vi "RB2 base station main 3.vi"() -> ()   [LabVIEW 2012]
uses:
  <vilib>/userdefined/High Color/IMAQdx.ctl
  <vilib>/vision/driver/NI_Vision_Acquisition_Software.lvlib
panel:
  out "Running?":bool
  out "All found?":bool
  in  "Data sent":string
  out "error out":errorcluster
  out "Image":T1(plugin-control)
  in  "stop":bool
  in  "Session In":T2="cam0"
  # "The Point Grey camera settings should be:\nAuto Exposure      Auto\nBrightness             Auto\nGain                       Auto\nFrame Rate           Auto\nShutter                  Auto\n\nThese values are programmed into this VI"
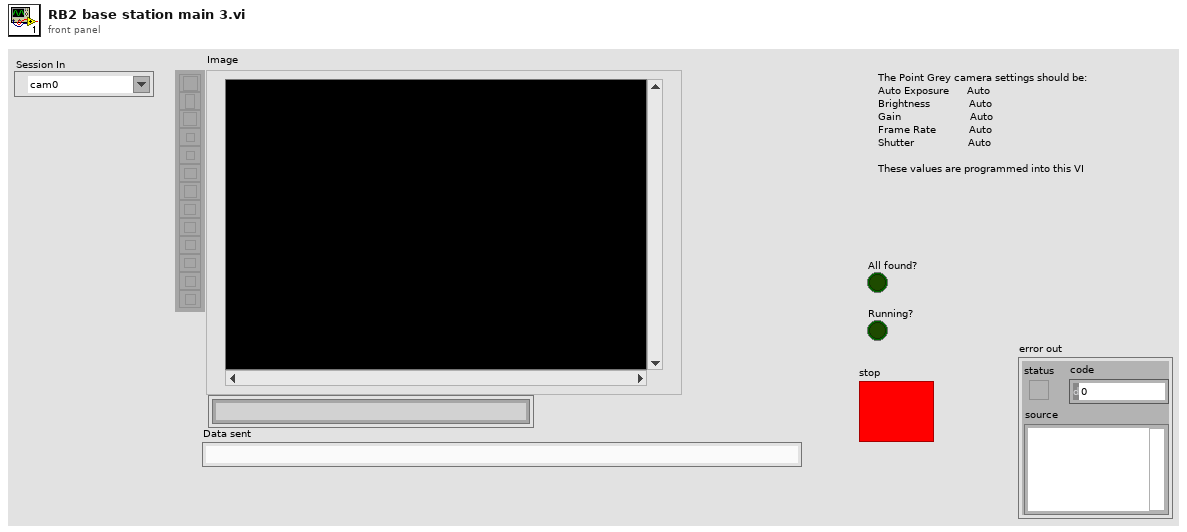
[diagram p1: front panel]
types:
  T1 = typedef "IMAQ Image.ctl" = refnum<image>
  T2 = typedef "IMAQdx.ctl" = refnum<k21>
  T3 = typedef "Image Type" = u32
  T4 = cluster{"String":string, "Pos. X":i32, "Pos. Y":i32, bool}[]
  T5 = cluster{"Pos. X":i32, "Pos. Y":i32, "Radius":i32, "Core Area":i32}[]
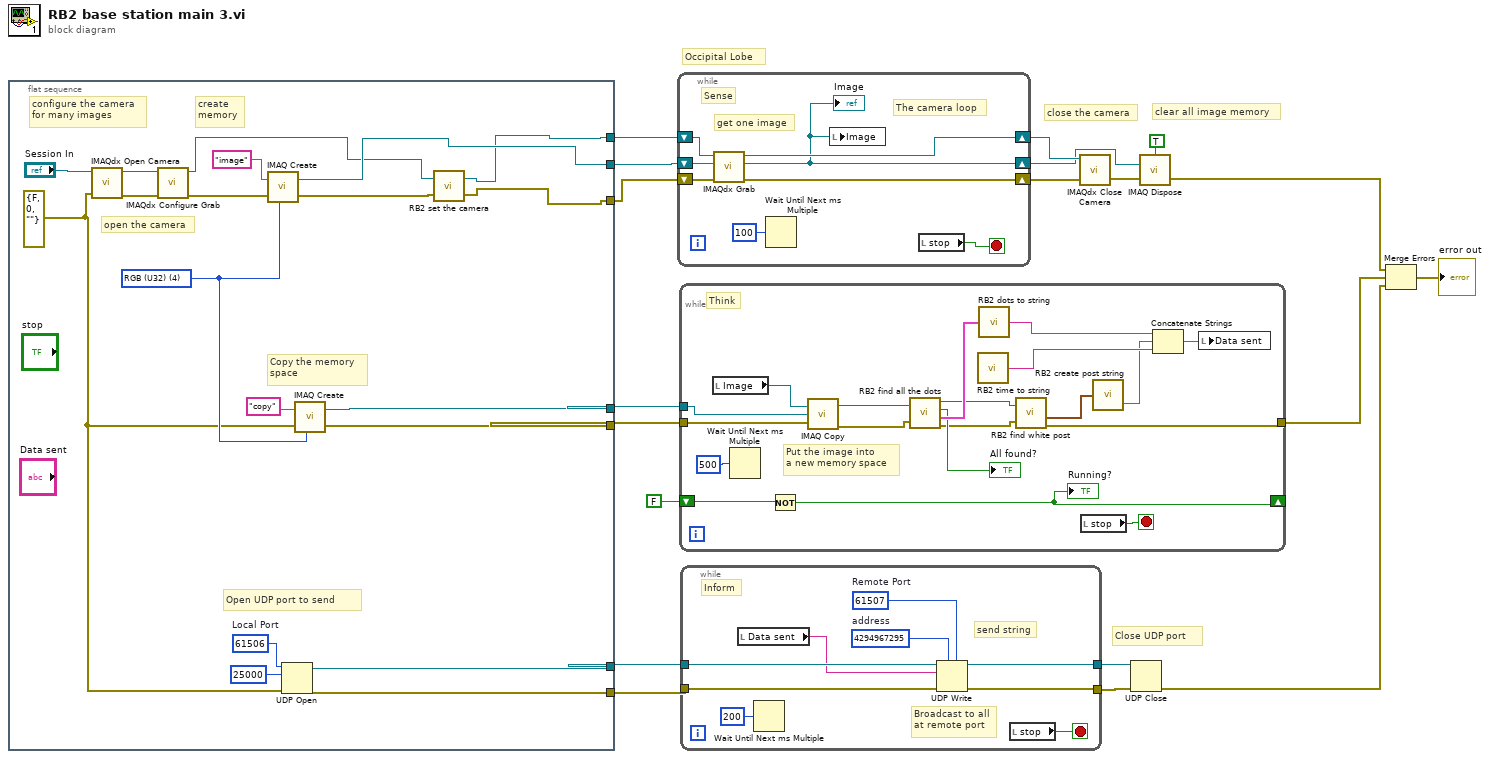
[diagram p0: block diagram]
diagram:
  # "Occipital Lobe"
  # "Close UDP port"
  # "clear all image memory"
  # "close the camera"
  n1 = flat-sequence {
    tunnel: [w22] -> w12
    tunnel: [w21] -> w13
    tunnel: [w24] -> w14
    tunnel: [w31] -> w10
    tunnel: [w30] -> w11
    tunnel: [w27] -> w4
    tunnel: [w26] -> w3
    frame #0 {
      w32 = T3 4 items=["Grayscale (U8)", "Grayscale (I16)", "Grayscale (SGL)", "Complex (CSG)", "RGB (U32)", "HSL (U32)", "RGB (U64)", "Grayscale (U16)"] ("Image Type")
      w29 = u16 61506  # Local Port
      w25 = errorcluster {"status"=FALSE, "code"=0, "source"=""} ("error in")
      # "Open UDP port to send"
      # "Copy the memory\nspace"
      # "create\nmemory"
      # "configure the camera\nfor many images"
      # "open the camera"
      n2 = call <vilib>:"IMAQdx Open Camera.vi"("error in"=w25, "Session In"="Session In") -> ("error out"=w36:errorcluster, "Session Out"=w37:T2)  [unwired: 1 in, 7 out]
      n3 = call <vilib>:"IMAQdx Configure Grab.vi"("error in"=w36, "Session In"=w37) -> ("error out"=w38:errorcluster, "Session Out"=w20:T2)  [unwired: 8 out]
      n4 = call "IMAQ Create"("Image Name"="image", "Image Type"=w32, "error in (no error)"=w38) -> ("New Image"=w24:T1, "error out"=w23:errorcluster)  [unwired: 1 in, 1 out]
      n5 = UDP Open(8:w25, 9:25000 ("timeout ms (25000)"), 11:w29) -> (port=w26:refnum<k16>, 0:w27:errorcluster)  [unwired: 3 out]
      n6 = call "IMAQ Create"("Image Name"="copy", "Image Type"=w32, "error in (no error)"=w25) -> ("New Image"=w30:T1, "error out"=w31:errorcluster)  [unwired: 2 in]
      n7 = call "RB2 set the camera.vi"("error in"=w23, "IMAQdx Session input"=w20) -> ("error out"=w22:errorcluster, "IMAQdx Session output"=w21:T2)
    }
  }
  n8 = while {
    shift-right: [w43] -> w19
    shift-left: w13 -> [w46]
    shift-right: [w39] -> w16
    shift-left: w14 -> [w45]
    shift-right: [w42] -> w18
    shift-left: w12 -> [w44]
    stop <- w40 stop-if-true
    # "Sense"
    # "The camera loop"
    # "get one image"
    n9 = call <vilib>:"IMAQdx Grab.vi"("error in"=w44, "Image In"=w45, "Session In"=w46) -> ("error out"=w42:errorcluster, "Image Out"=w39:T1, "Session Out"=w43:T2)  [unwired: 5 in, 1 out]
    "Image" <- w39
    n10 = Wait Until Next ms Multiple(millisecond multiple=u32 100) -> ()  [unwired: 1 out]
    n11 = local write "Image"(w39) -> ()
    n12 = local read "stop"() -> (w40:bool)
  }
  n13 = while {
    tunnel: w11 -> [w64]
    tunnel: w10 -> [w65]
    tunnel: [w50] -> w8
    shift-right: [w59] -> _
    shift-left: FALSE -> [w60]
    stop <- w62 stop-if-true
    # "Think"
    # "Put the image into \na new memory space"
    n14 = local read "Image"() -> (w63:T1)
    n15 = Wait Until Next ms Multiple(millisecond multiple=u32 500) -> ()  [unwired: 1 out]
    n16 = Not(x=w60) -> (.not. x?=w59:bool)
    "Running?" <- w59
    n17 = call "IMAQ Copy"("error in (no error)"=w65, "Image Dst"=w64, "Image Src"=w63) -> ("error out"=w55:errorcluster, "Image Dst Out"=w56:T1)  [unwired: 3 in]
    n18 = call "RB2 find all the dots.vi"("Image In"=w56, "error in"=w55) -> ("Image Out"=w51:T1, "All Found?"=→"All found?":bool, "Dot Array"=w57:T4, "error out"=w52:errorcluster)
    n19 = call "RB2 time to string.vi"() -> ("time string"=w48:string)  [unwired: 1 in]
    n20 = call "RB2 dots to string.vi"("Dot Array"=w57) -> ("dot location string"=w58:string)
    n21 = call "RB2 find white post.vi"("Image In"=w51, "error in"=w52) -> ("White dot\nLocation"=w49:T5, "error out"=w50:errorcluster)  [unwired: 2 out]
    n22 = local read "stop"() -> (w62:bool)
    n23 = call "RB2 create post string.vi"("White dot\nLocation"=w49) -> ("Post String"=w47:string)  [unwired: 1 out]
    n24 = Concatenate Strings(w58, w47, w48) -> (w53:string)
    n25 = local write "Data sent"(w53) -> ()
  }
  n26 = while {
    tunnel: w3 -> [w74]
    tunnel: w4 -> [w73]
    tunnel: [w72] -> w6
    tunnel: [w71] -> w5
    stop <- w67 stop-if-true
    w70 = u16 61507  # Remote Port
    w69 = u32 4294967295  # address
    # "Inform"
    # "send string"
    # "Broadcast to all\nat remote port"
    n27 = local read "Data sent"() -> (w68:string)
    n28 = Wait Until Next ms Multiple(millisecond multiple=u32 200) -> ()  [unwired: 1 out]
    n29 = UDP Write(address=w69, port or service name=w70, connection ID=w74, data in=w68, 8:w73) -> (error out=w72:errorcluster, 3:w71:refnum<k16>)  [unwired: 1 out]
    n30 = local read "stop"() -> (w67:bool)
  }
  n31 = call <vilib>:"IMAQdx Close Camera.vi"("error in"=w18, "Session In"=w19) -> ("error out"=w17:errorcluster)  [unwired: 9 out]
  n32 = UDP Close(connection ID=w5, 8:w6) -> (error out=w2:errorcluster)  [unwired: 1 out]
  n33 = call "IMAQ Dispose"("All Images? (No)"=TRUE, "Image"=w16, "error in (no error)"=w17) -> ("error out"=w9:errorcluster)  [unwired: 3 out]
  n34 = Merge Errors(w9, w8, w2) -> (→"error out":errorcluster)
